vi "Create Bus Load Calculator.vi"   [LabVIEW 2019, in "XNET-Bus-Load-Calculator.lvlib"]
uses:
  XNET-Bus-Load-Calculator.lvlib
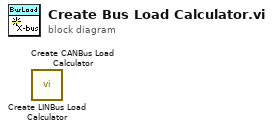
[diagram p0: block diagram]
diagram:
  n1 = call "Create LINBus Load Calculator.vi"() -> ()  [unwired: 10 in, 2 out]
  n2 = call "Create CANBus Load Calculator.vi"() -> ()  [unwired: 10 in, 2 out]
